vi "Speed Config Global.vi"(0 "Speed Settings In":T1={"max window"=1400.0, "min window"=45.0, "CommSegments"=2.0}, 2 "Mode (Read)":T2(ring), 7 "Controller In":bool, 11 "Speed Enable In":bool[](array[boolean])) -> (4 "Speed Settings Out":T1={"max window"=1400.0, "min window"=45.0, "CommSegments"=2.0}, 8 "Controller Out":bool, 15 "Speed Enable Out":bool[](array[boolean]))   [LabVIEW 2013]
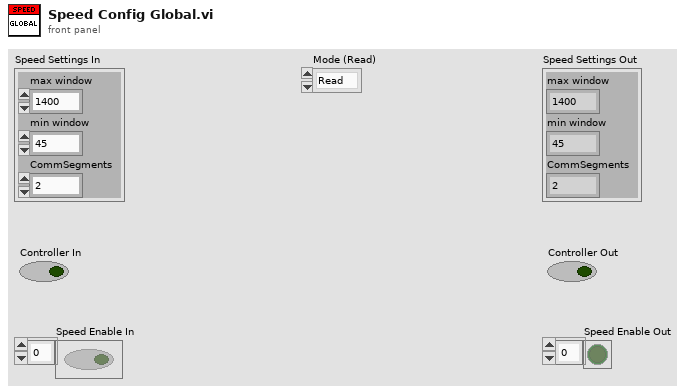
[diagram p1: front panel]
types:
  T1 = cluster{"max window":dbl, "min window":dbl, "CommSegments":dbl}
  T2 = enum16{"Read", "Write Settings", "Write Enables"}
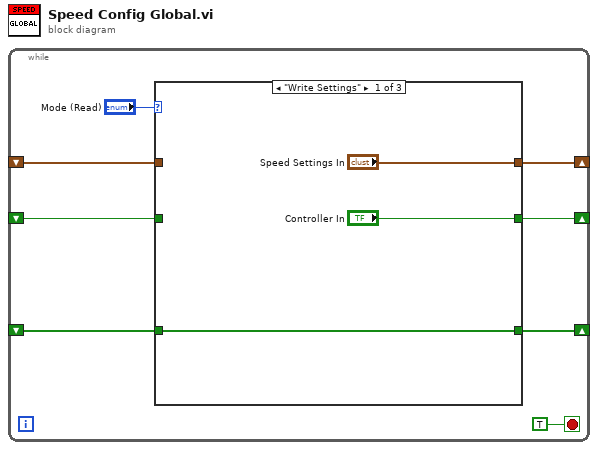
[diagram p0: block diagram]
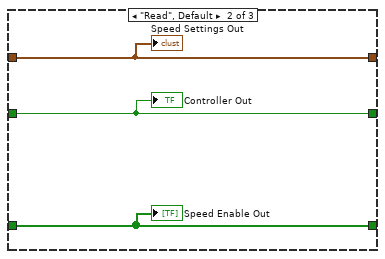
[diagram p2: hidden frame]
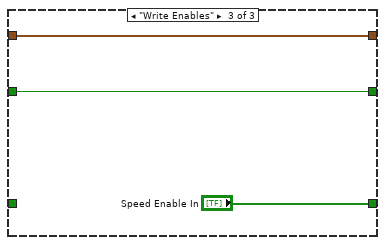
[diagram p3: hidden frame]
diagram:
  n1 = while {
    shift-right: [w6] -> _
    shift-left: _ -> [w5]
    shift-right: [w4] -> _
    shift-left: _ -> [w3]
    shift-right: [w2] -> _
    shift-left: _ -> [w1]
    stop <- TRUE stop-if-true
    n2 = case shown="\"Write Settings\"" "Mode (Read)" {
      tunnel: ["Speed Settings In" w13 w15] -> w6
      tunnel: w5 -> [_ w13 w15]
      tunnel: ["Controller In" w12 w16] -> w4
      tunnel: w3 -> [_ w12 w16]
      tunnel: [w11 w14 "Speed Enable In"] -> w2
      tunnel: w1 -> [w11 w14 _]
      frame "Write Settings" {
      }
      frame "Read", Default {
        "Speed Enable Out" <- w14
        "Speed Settings Out" <- w13
        "Controller Out" <- w12
      }
      frame "Write Enables" {
      }
    }
  }
